vi "RT_Convert_Bulk.vi"() -> ()   [LabVIEW 2022 SP3]
panel:
  in  "file ext":string="*.eye"
  in  "Use Selected Files":bool
  in  "Listbox":i32[](listbox)
  in  "Choose Directory":path
  out "Comment":string
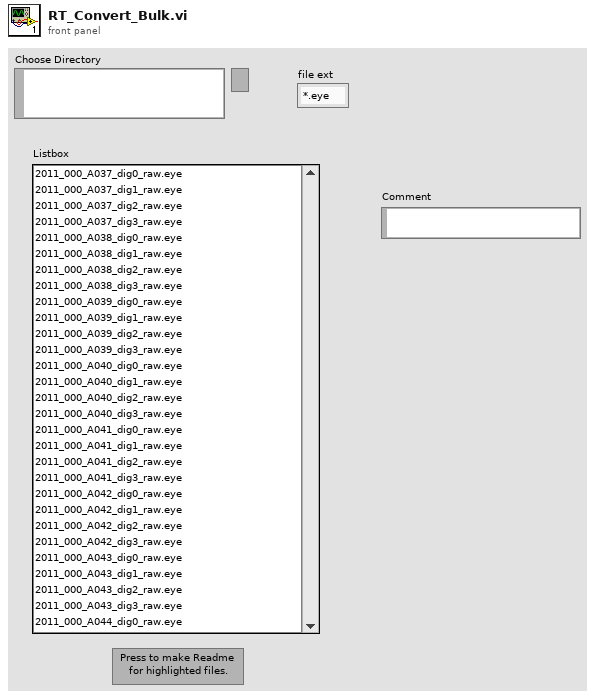
[diagram p1: front panel]
types:
  T1 = typedef "Header.ctl" = cluster{"header info":cluster{"Header":string, "Head length":i16}, "A/D info":cluster{"# rf points per line":u16, "# lines per scan":u16, "sample rate MHz":u16, "# A/D bits":i16, "# bytes per A/D":u16, "TGC Flag":u16, "A/D Type":string}, "Tranducer Info":cluster{"bandwidth":sgl, "center freq":sgl, "start freq":sgl, "ID":i32}, "Scan Info":cluster{"delay":sgl, "pivot distance":sgl, "sector scan angle":sgl, "operator":string, "Scan Mode":string, "location":string}, "Time/Date Info":cluster{"date":string, "time":string}, "RF Info":cluster{"RF file name":string, "RF file att":string, "RF cal file name":string, "RF cal file att":string}, "Patient Info":cluster{"ID":string, "extended ID":string, "age":u16, "sex":string, "previously\nscanned":string, "PSA":sgl, "LOS":u8, "Ethnicty 2":u8, "Race":u8}, "Tissue Type":cluster{"organ":i16, "disease type":i16, "disease location":i16, "IQ_pts":u16, "RcvBuffer":u8, "RcvFrame":u16, "IQBuff":u8, "IQFrame":u16, "IQPage":u8}, "Votage scaling":cluster{"Digitizer (dB)":sgl, "Gain (dB)":sgl, "Atten (dB)":sgl}, "Comment":string, "Misc Info":cluster{"avg num":u16, "c speed":i16, "Div By or SF zones":i16, "XMIT CHS":u8, "RCV CHS":u8, "Xmit angle":sgl}, "Therapy Parameters":cluster{"Theraputic Freq (MHz)":sgl, "Time on (s)":sgl, "Therapy amplitude (mV)":sgl, "Lines Before":u16, "Lines After":u16}, "Scan Settings":cluster{"Energy (uJ or V)":u8, "Damp (Ohm) or Fc":u8, "HP Filt (KHz)":u8, "LP Filt (MHz)":u8, "Gain (db)":u8, "prf (kHz)":sgl, "Distance between\nscan lines (um)":u16, "Distance between\nscan planes (um)":u16, "Scan line gap (um)":sgl, "Scan plane gap (um)":sgl}, "Compression Parameters":cluster{"F1 (MHz)":sgl, "F2 (MHz)":sgl, "% taper":sgl, "duration":sgl}, "Patient Info Xtra":cluster{"First Name":string, "Last Name":string, "Notes":string}, "ROI Box":u16[]}
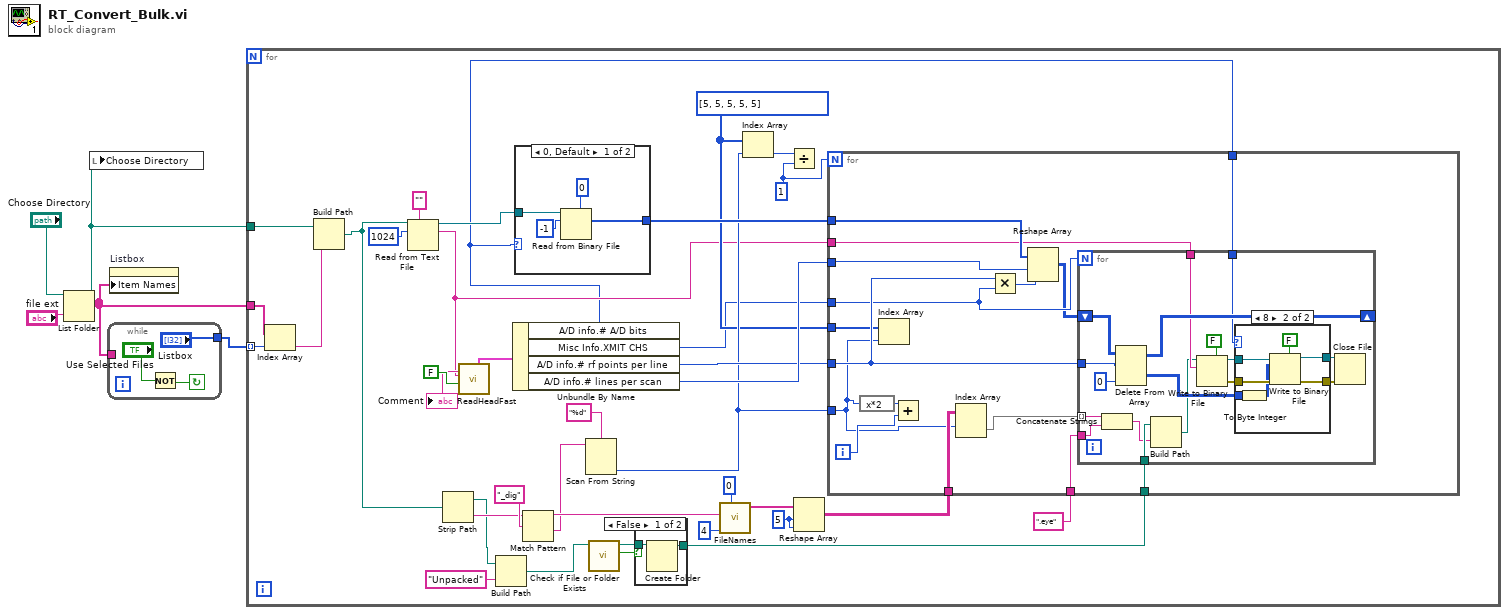
[diagram p0: block diagram]
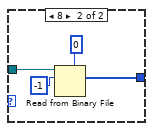
[diagram p2: hidden frame]
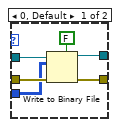
[diagram p4: hidden frame]
diagram:
  n1 = List Folder(path="Choose Directory", pattern="file ext") -> (path out=w3:path, filenames=w2:string[])  [unwired: 1 in, 3 out]
  n2 = local write "Choose Directory"(w3) -> ()
  n3 = while {
    tunnel: ["Listbox"] -> w1
    tunnel: w2 -> [_]
    stop <- w8 continue-if-true
    n4 = Not(x="Use Selected Files") -> (.not. x?=w8:bool)
  }
  n5 = property on="Listbox" class="LstBox (strict)"("Item Names"=w2) -> ()  [unwired: 2 in, 2 out]
  n6 = for {
    tunnel: w3 -> [w21]
    tunnel: w2 -> [w23]
    tunnel: w1 -> [w22] mode=indexing
    w19 = 1
    w34 = 5 ("dimension size")
    w29 = i32[] [5, 5, 5, 5, 5]
    n7 = Index Array(array=w23, index=w22) -> (element=w24:string)
    n8 = Build Path(base path=w21, name or relative path=w24) -> (appended path=w20:path)
    n9 = Read from Text File(prompt (Open existing file)="", file (use dialog)=w20, count=1024) -> (refnum out=w39:refnum<file>, text=w27:string)  [unwired: 1 in, 2 out]
    n10 = Strip Path(path=w20) -> (stripped path=w15:path, name=w17:string)
    n11 = call "ReadHeadFast.vi"("Use File?"=FALSE, "raw reader"=w27) -> ("Header In"=w43:T1, "raw header out"=→"Comment":string)  [unwired: 6 in, 2 out]
    n12 = Build Path(base path=w15, name or relative path="Unpacked") -> (appended path=w12:path)
    n13 = Unbundle By Name(w43) -> ("A/D info.# A/D bits"=w9:i16, "Misc Info.XMIT CHS"=w18:u8, "A/D info.# rf points per line"=w41:u16, "A/D info.# lines per scan"=w42:u16)
    n14 = case shown="0, Default" w9 {
      tunnel: [w50 w54] -> w40
      tunnel: w39 -> [w49 w53]
      frame 0, Default {
        n15 = Read from Binary File(5:i16 0, 10:-1 ("count (1)"), 11:w49) -> (2:w50:i16[])  [unwired: 3 in, 3 out]
      }
      frame 8 {
        n16 = Read from Binary File(5:i8 0, 10:-1 ("count (1)"), 11:w53) -> (2:w54:i8[])  [unwired: 3 in, 3 out]
      }
    }
    n17 = Match Pattern(string=w17, regular expression="_dig") -> (before substring=w36:string, after substring=w16:string)  [unwired: 1 in, 2 out]
    n18 = Scan From String(format string="%d", input string=w16) -> (output 1=w30:i32)  [unwired: 3 in, 3 out]
    n19 = call <vilib>:"Check if File or Folder Exists.vi"("path"=w12) -> ("file or folder exists?"=w10:bool, "dup path"=w11:path)  [unwired: 8 in, 1 out]
    n20 = case shown="False" w10 {
      tunnel: [w56 w57] -> w13
      tunnel: w11 -> [w55 w57]
      frame False {
        n21 = Create Folder(path (use dialog)=w55) -> (created path=w56:path)  [unwired: 2 in, 2 out]
      }
      frame True {
      }
    }
    n22 = call "FileNames.vi"("Digits"=0, "Dig Config"=4, "Scan Name"=w36) -> ("All files"=w35:string[])  [unwired: 4 in, 4 out]
    n23 = Index Array(array=w29, index=w30) -> (element=w28:i32)
    n24 = Divide(x=w28, y=w19) -> ()  [unwired: 1 out]
    n25 = Reshape Array(w35, w34, w34) -> (w26:string[][])
    n26 = for {
      N: w19 -> [_]
      tunnel: w29 -> [w69]
      tunnel: w40 -> [w72]
      tunnel: w42 -> [w71]
      tunnel: w41 -> [w70]
      tunnel: w30 -> [w60]
      tunnel: w26 -> [w68]
      tunnel: w27 -> [w64]
      tunnel: w13 -> [w63]
      tunnel: ".eye" ("regular expression") -> [w62]
      tunnel: w18 -> [w61]
      tunnel: w9 -> [w58]
      i -> [w65]
      n27 = expression code="x*2"(w60) -> (w66:i32)
      n28 = Index Array(array=w69, index=w60) -> ()  [unwired: 1 out]
      n29 = Add(x=w66, y=w65) -> ()  [unwired: 1 out]
      n30 = Index Array(array=w68, index (row)=w60) -> (element=w67:string[])  [unwired: 1 in]
      n31 = Multiply(x=w70, y=w61) -> (x*y=w73:u16)
      n32 = Reshape Array(w72, w71, w73) -> (w59:i16[][])
      n33 = for {
        N: w61 -> [_]
        shift-right: [w88] -> _
        shift-left: w59 -> [w90]
        tunnel: w70 -> [w87]
        tunnel: w67 -> [w77] mode=indexing
        tunnel: w64 -> [w80]
        tunnel: w63 -> [w79]
        tunnel: w62 -> [w75]
        tunnel: w58 -> [w74]
        n34 = Concatenate Strings(w77, w75) -> (w76:string)
        n35 = Delete From Array(array=w90, length=w87, index (col)=0 ("disabled index (col)")) -> (deleted portion=w81:i16[][], array with subset deleted=w88:i16[][])  [unwired: 1 in]
        n36 = Build Path(base path=w79, name or relative path=w76) -> (appended path=w78:path)
        n37 = Write to Binary File(file (use dialog)=w78, data=w80, 5:FALSE ("prepend array or string size? (T)")) -> (refnum out=w85:refnum<file>, error out=w86:errorcluster)  [unwired: 3 in, 1 out]
        n38 = case shown="8" w74 {
          tunnel: w86 -> [w96 w103]
          tunnel: w85 -> [w95 w102]
          tunnel: [w94 w101] -> w84
          tunnel: [w93 w100] -> w83
          tunnel: w81 -> [w91 w98]
          frame 0, Default {
            n39 = Write to Binary File(file (use dialog)=w95, data=w91, error in=w96, 5:FALSE ("prepend array or string size? (T)")) -> (refnum out=w93:refnum<file>, error out=w94:errorcluster)  [unwired: 2 in, 1 out]
          }
          frame 8 {
            n40 = To Byte Integer(number=w98) -> (8bit integer=w97:i8[][])
            n41 = Write to Binary File(file (use dialog)=w102, data=w97, error in=w103, 5:FALSE ("prepend array or string size? (T)")) -> (refnum out=w100:refnum<file>, error out=w101:errorcluster)  [unwired: 2 in, 1 out]
          }
        }
        n42 = Close File(refnum=w83, error in=w84) -> ()  [unwired: 2 out]
      }
    }
  }
